vi "Cal10-WriteOutCurrentSetup.vi"(11 "CalibrationPath":path) -> (3 "String":string)   [LabVIEW 2016]
uses:
  Anemometry Sub Vis/File/Setup_Filetype.ctl
  Anemometry Sub Vis/Globals/Calib_global.vi
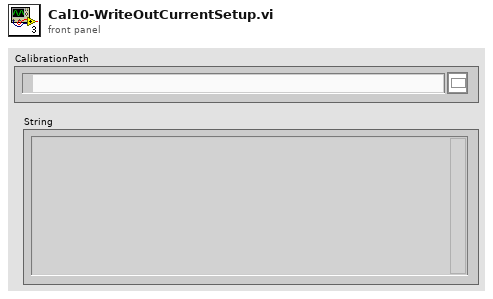
[diagram p1: front panel]
types:
  T1 = typedef "Setup_Filetype.ctl" = enum16{"Measurement Setups", "Calibration Setups", "General", "Results File Plotter Setups", "Speed Calib Tweaks"}
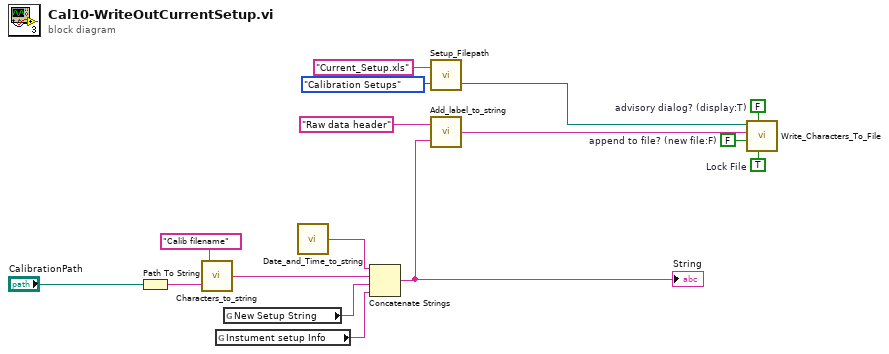
[diagram p0: block diagram]
diagram:
  w11 = TRUE  # Lock File
  w5 = FALSE  # advisory dialog? (display:T)
  w4 = FALSE  # append to file? (new file:F)
  n1 = Path To String(path="CalibrationPath") -> (string=w10:string)
  n2 = call "Characters_to_string.vi"("Characters to write"=w10, "Label for characters"="Calib filename") -> ("Output string"=w1:string)
  n3 = global read "Calib_global.vi" "Instument setup Info"() -> (w9:string)
  n4 = global read "Calib_global.vi" "New Setup String"() -> (w8:string)
  n5 = call "Date_and_Time_to_string.vi"() -> ("Date and time (spreadsheet)"=w2:string)
  n6 = Concatenate Strings(w2, w1, w8, w9) -> (w13:string)
  "String" <- w13
  n7 = call "Setup_Filepath.vi"("Setup File Type"=Setup_Filetype."Calibration Setups", "Filename in"="Current_Setup.xls") -> ("Filename Out"=w16:path)  [unwired: 1 out]
  n8 = call "Add_label_to_string.vi"("String to write"=w13, "File Label"="Raw data header") -> ("Output string"=w7:string)
  n9 = call "Write_Characters_To_File.vi"("file path (dialog if empty)"=w16, "advisory dialog? (display:T)"=w5, "character string"=w7, "append to file? (new file:F)"=w4, "Lock File"=w11) -> ()  [unwired: 4 out]
